vi "uMsg unDefer Reply.vi"(8 "error in (no error)":errorcluster, 11 "uMsg in":refnum<class "uMsg.lvclass">) -> (0 "error out":errorcluster, 3 "uMsg out":refnum<class "uMsg.lvclass">)   [LabVIEW 2021, in "uFramework.lvlib" / "uMsg.lvclass"]
doc: "Set the flag to send out the reply to sender when the \"Send reply\" message is called."
uses:
  uMsg.lvclass
  uMsg.lvclass/uMsg.ctl
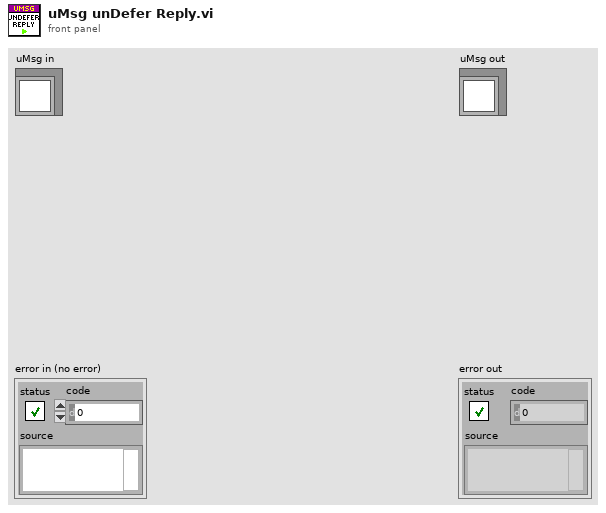
[diagram p1: front panel]
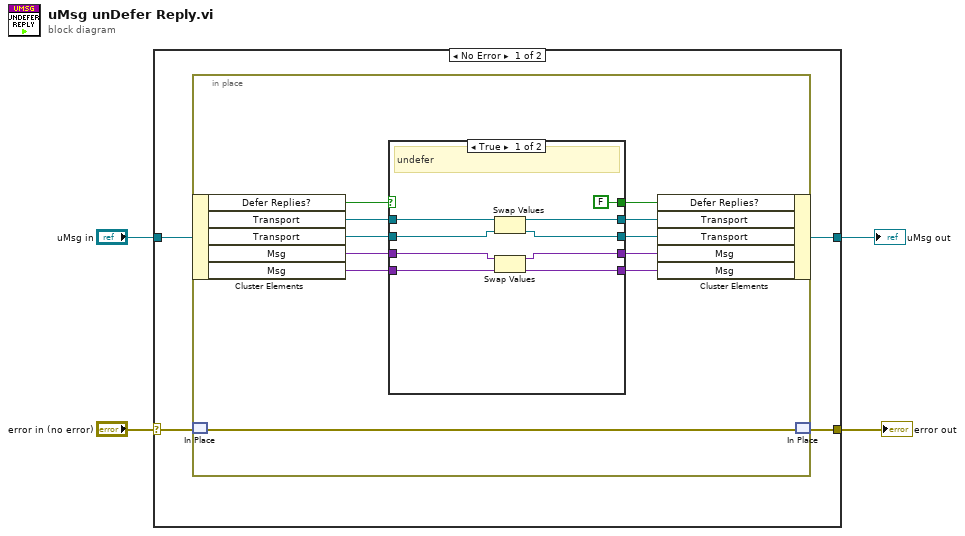
[diagram p0: block diagram]
diagram:
  n1 = case shown="No Error" "error in (no error)" {
    selector: "error in (no error)" -> [w8 w34]
    tunnel: [w7 w34] -> w3
    tunnel: [w5 w35] -> w2
    tunnel: "uMsg in" -> [w6 w35]
    frame No Error {
      n2 = in-place {
        n3 = in-place-cluster #1(w6) -> ("Defer Replies?"=w18:bool, "Transport"=w13:refnum<class "uTransport.lvclass">, "Transport"=w14:refnum<class "uTransport.lvclass">, "Msg"=w15:variant, "Msg"=w16:variant)
        n4 = in-place-match #2(w8) -> (w19:errorcluster)
        n5 = case shown="True" w18 {
          selector: w18 -> [_ w33]
          tunnel: [FALSE w33] -> w17
          tunnel: w16 -> [w23 w29]
          tunnel: w15 -> [w20 w30]
          tunnel: w14 -> [w26 w31]
          tunnel: w13 -> [w27 w32]
          tunnel: [w25 w32] -> w12
          tunnel: [w24 w31] -> w11
          tunnel: [w21 w30] -> w10
          tunnel: [w22 w29] -> w9
          frame True {
            # "undefer"
            n6 = Swap Values(12:w27, 14:w26) -> (1:w25:refnum<class "uTransport.lvclass">, 3:w24:refnum<class "uTransport.lvclass">)  [unwired: 1 in]
            n7 = Swap Values(12:w20, 14:w23) -> (1:w21:variant, 3:w22:variant)  [unwired: 1 in]
          }
          frame False {
            # "Already undeferred"
          }
        }
        n8 = in-place-cluster #1("Defer Replies?"=w17, "Transport"=w12, "Transport"=w11, "Msg"=w10, "Msg"=w9) -> (w5:refnum<class "uMsg.lvclass">)
        n9 = in-place-match #2(w19) -> (w7:errorcluster)
      }
    }
    frame Error {
    }
  }
  "error out" <- w3
  "uMsg out" <- w2
